vi "TagValue-to-JSON.vi"(8 "error in (no error)":errorcluster, 10 "Value":string, 11 "Tag":string) -> (0 "error out":errorcluster, 3 "Command JSON string":string)   [LabVIEW 2023]
uses:
  Controls/tagValue.ctl
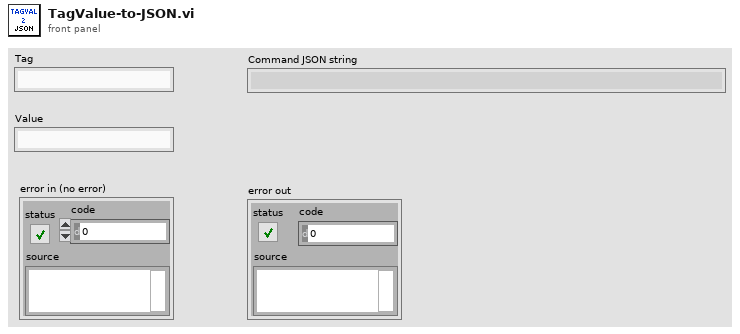
[diagram p1: front panel]
types:
  T1 = typedef "tagValue.ctl" = cluster{"type":string, "tag":string, "value":string, "t":string}
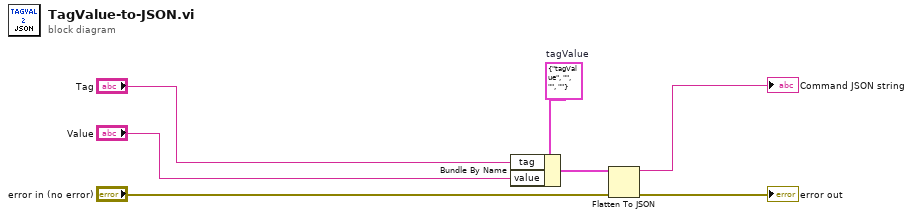
[diagram p0: block diagram]
diagram:
  w2 = T1 {"type"="tagValue", "tag"="", "value"="", "t"=""}  # tagValue
  n1 = Bundle By Name(cluster=w2, "tag"="Tag", "value"="Value") -> (w3:T1)
  n2 = Flatten To JSON(anything=w3, error in (no error)="error in (no error)") -> (JSON string=→"Command JSON string":string, 11:→"error out":errorcluster)  [unwired: 1 in]
